vi "User Input Dialog.vi"(7 "error in (no error)":errorcluster, 9 "Message title":string, 10 "Enable":bool=TRUE) -> (0 "error out":errorcluster, 1 "OK?":bool caption="OK", 3 "Message out":string)   [LabVIEW 2019]
doc: "Displays a standard dialog box that prompts users to enter information, such as a user name and password.\n--------------------\n\nThis Express VI is configured as follows:\n\nMessage to Display to the User:\nThe inputs are:"
panel:
  in  "Message":string
  in  "Cancel":bool
  in  "OK":bool caption="OK2"
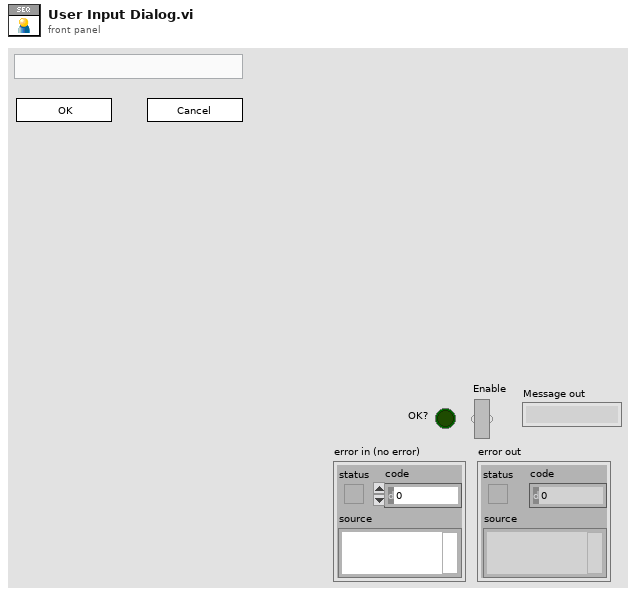
[diagram p1: front panel]
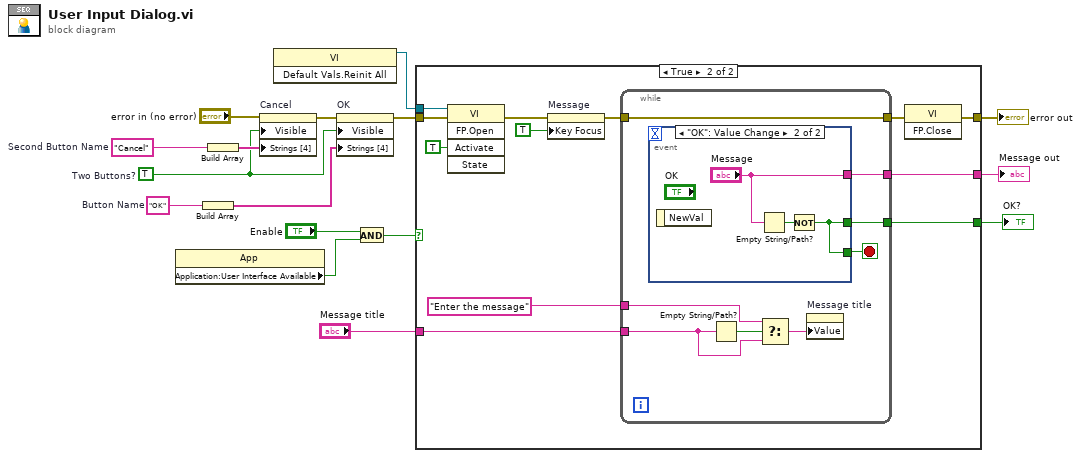
[diagram p0: block diagram]
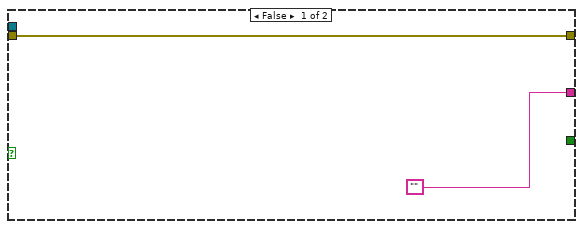
[diagram p2: hidden frame]
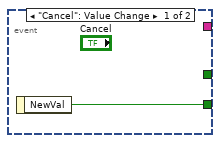
[diagram p3: hidden frame]
diagram:
  w13 = "Cancel"  # Second Button Name
  w11 = "OK"  # Button Name
  w2 = TRUE  # Two Buttons?
  n1 = property class="App"() -> ("Application:User Interface Available"=w8:bool)  [unwired: 2 in, 2 out]
  n2 = Build Array(w11) -> (w12:string[])
  n3 = Build Array(w13) -> (w14:string[])
  n4 = property on="Cancel" class="Bool"(error in="error in (no error)", "Visible"=w2, "Strings [4]"=w14) -> (error out=w15:errorcluster)  [unwired: 1 in, 1 out]
  n5 = invoke class="VI" method="Default Vals.Reinit All"() -> (reference out=w7:refnum<vi>)  [unwired: 3 in, 2 out]
  n6 = property on="OK" class="Bool"(error in=w15, "Visible"=w2, "Strings [4]"=w12) -> (error out=w5:errorcluster)  [unwired: 1 in, 1 out]
  n7 = And(x="Enable", y=w8) -> (x .and. y?=w6:bool)
  n8 = case shown="True" w6 {
    tunnel: [_ w30] -> w16
    tunnel: w5 -> [w18 w29]
    tunnel: [w18 w28] -> w10
    tunnel: w7 -> [_ w27]
    tunnel: ["" w24] -> w4
    tunnel: "Message title" -> [_ w23]
    frame False {
    }
    frame True {
      n9 = invoke class="VI" method="FP.Open"(reference=w27, error in=w29, "Activate"=TRUE ("Activate?")) -> (error out=w20:errorcluster)  [unwired: 2 in, 4 out]
      n10 = property on="Message" class="Str"(error in=w20, "Key Focus"=TRUE) -> (error out=w19:errorcluster)  [unwired: 1 in, 1 out]
      n11 = while "Main While Loop" {
        tunnel: [w36] -> w30
        tunnel: w19 -> [w38]
        tunnel: [w38] -> w25
        tunnel: [w35] -> w24
        tunnel: w23 -> [w31]
        tunnel: "Enter the message" ("Message title") -> [w33]
        stop <- w37 stop-if-true
        n12 = event shown="[1] \"OK\": Value Change" {
          selector: _ -> [_ _]
          dyn-events: _ -> [_ _]
          timeout: _ -> [_ _]
          tunnel: [w39 w40] -> w37
          tunnel: [_ w40] -> w36
          tunnel: [_ "Message"] -> w35
          event "Cancel": Value Change {
            n13 = event-data() -> ("NewVal"=w39:bool)  [unwired: 1 in]
          }
          event "OK": Value Change {
            n14 = event-data() -> ()  [unwired: 1 in, 1 out]
            n15 = Empty String/Path?(string/path="Message") -> (empty?=w41:bool)
            n16 = Not(x=w41) -> (.not. x?=w40:bool)
          }
        }
        n17 = Empty String/Path?(string/path=w31) -> (empty?=w34:bool)
        n18 = Select(t=w33, s=w34, f=w31) -> (s? t:f=w32:string)
        n19 = property on="Message title" class="Str"("Value"=w32) -> ()  [unwired: 2 in, 2 out]
      }
      n20 = invoke class="VI" method="FP.Close"(error in=w25) -> (error out=w28:errorcluster)  [unwired: 2 in, 2 out]
    }
  }
  "OK?" <- w16
  "error out" <- w10
  "Message out" <- w4
